vi "Calculate Restarts.vi"(0 "Restarts Cluster":T3={"CMD Starts:"=[0, 0, 0, 0, 0, 0], "Restarts:"=[0, 0, 0, 0, 0, 0], "Total CMD:"=[0, 0, 0, 0, 0, 0], "Total Restarts:"=[0, 0, 0, 0, 0, 0]}, 5 "Restarts Limits":T1={"High Limits:"=[30, 30, 30, 30, 30, 30], "Low Limits:"=[30, 30, 30, 30, 30, 30]}, 7 "Run Profile":bool, 9 "Actual Starts":T2={"Actual Pump Starts"=[0, 0, 0, 0, 0, 0], "Initial Actual Starts"=[0, 0, 0, 0, 0, 0], "Tot Act Starts"=[0, 0, 0, 0, 0, 0], "Tot Init Act Starts"=[0, 0, 0, 0, 0, 0]}, 11 "Actual Pump Starts (FPGA)":u32[](array[numeric])=[0, 0, 0, 0, 0, 0]) -> (4 "Restarts Cluster OUT":T3, 6 "Restarts Alarm":bool, 8 "Restarts Limits OUT":T1={"High Limits:"=[30, 30, 30, 30, 30, 30], "Low Limits:"=[30, 30, 30, 30, 30, 30]}, 10 "Actual Starts OUT":T2)   [LabVIEW 2019]
uses:
  Type Defs/Restarts Cluster.ctl
  Type Defs/Restarts Limits.ctl
  Type Defs/Actual Starts.ctl
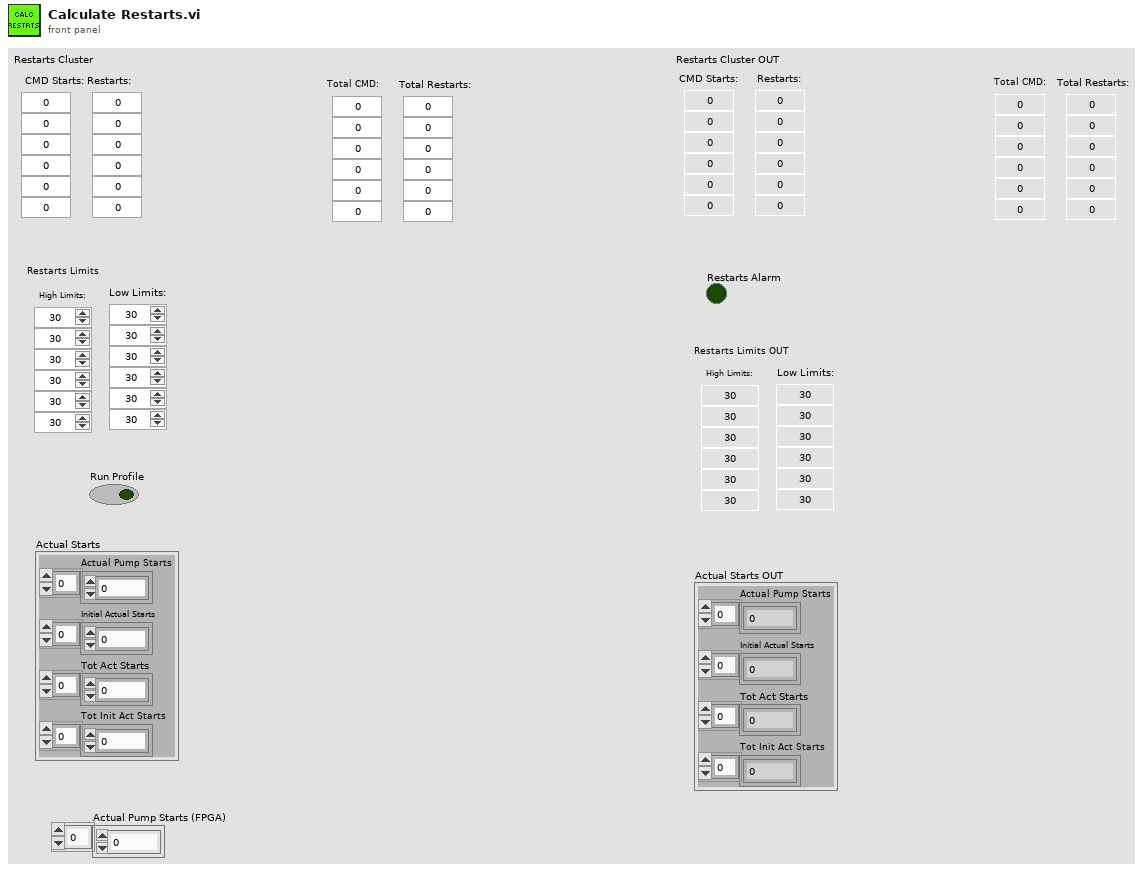
[diagram p1: front panel]
types:
  T1 = typedef "Restarts Limits.ctl" = cluster{"High Limits:":i32[], "Low Limits:":i32[]}
  T2 = typedef "Actual Starts.ctl" = cluster{"Actual Pump Starts":i32[], "Initial Actual Starts":i32[], "Tot Act Starts":i32[], "Tot Init Act Starts":i32[]}
  T3 = typedef "Restarts Cluster.ctl" = cluster{"CMD Starts:":i32[], "Restarts:":i32[], "Total CMD:":i32[], "Total Restarts:":i32[]}
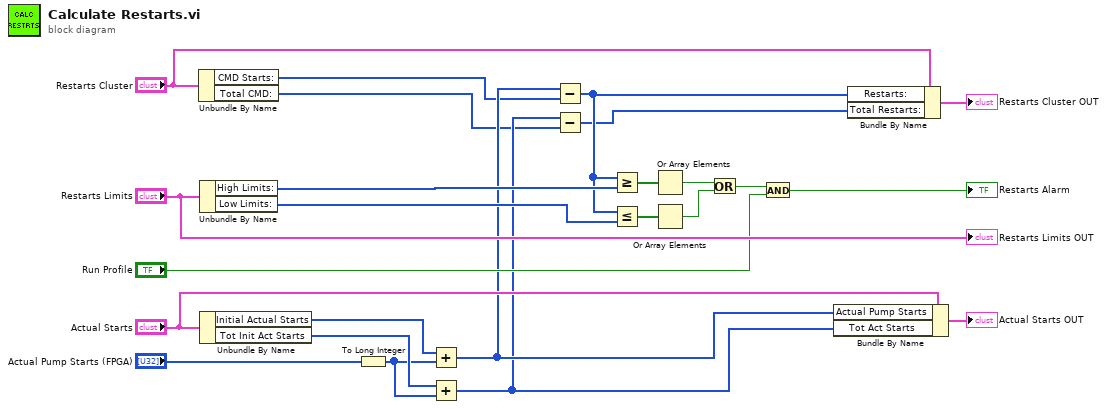
[diagram p0: block diagram]
diagram:
  n1 = Unbundle By Name("Restarts Cluster") -> ("CMD Starts:"=w4:i32[], "Total CMD:"=w2:i32[])
  n2 = Unbundle By Name("Restarts Limits") -> ("High Limits:"=w18:i32[], "Low Limits:"=w17:i32[])
  n3 = Unbundle By Name("Actual Starts") -> ("Initial Actual Starts"=w12:i32[], "Tot Init Act Starts"=w6:i32[])
  n4 = To Long Integer(number="Actual Pump Starts (FPGA)") -> (32bit integer=w5:i32[])
  n5 = Add(x=w12, y=w5) -> (x+y=w10:i32[])
  n6 = Add(x=w6, y=w5) -> (x+y=w3:i32[])
  n7 = Subtract(x=w10, y=w4) -> (x-y=w15:i32[])
  n8 = Subtract(x=w3, y=w2) -> (x-y=w1:i32[])
  n9 = Greater Or Equal?(x=w15, y=w18) -> (x >= y?=w20:bool[])
  n10 = Less Or Equal?(x=w15, y=w17) -> (x <= y?=w21:bool[])
  n11 = Or Array Elements(Boolean array=w20) -> (logical OR=w22:bool)
  n12 = Or Array Elements(Boolean array=w21) -> (logical OR=w23:bool)
  n13 = Or(x=w22, y=w23) -> (x .or. y?=w24:bool)
  n14 = And(x=w24, y="Run Profile") -> (x .and. y?=→"Restarts Alarm":bool)
  n15 = Bundle By Name(cluster="Actual Starts", "Actual Pump Starts"=w10, "Tot Act Starts"=w3) -> (→"Actual Starts OUT":T2)
  n16 = Bundle By Name(cluster="Restarts Cluster", "Restarts:"=w15, "Total Restarts:"=w1) -> (→"Restarts Cluster OUT":T3)
  "Restarts Limits OUT" <- "Restarts Limits"
